vi "ClawGetStatus.vi"(8 "error in (no error)":errorcluster, 11 "MotorControlDevRef":T1={"DeviceStatus"={"status"=FALSE, "code"=0, "source"=""}, "Type"=enum."PWM", "PWM"={"Controller"=enum."Controller 1", "PWM Channel"=enum."PWM 1", "DeadBand"={"Name"="", "maxPositivePwm"=0, "minPositivePwm"=0, "centerPwm"=0, "maxNegativePwm"=0, "minNegativePwm"=0, "angularRange"=0}}, "CAN"={"Device Number"=0, "Control Mode"=enum."Percent VBus", "Semaphore"=refnum, "Max Vout"=12.0, "TalonSRX Control Mode"=enum."Percent VBus"}, "Invert"=FALSE, "TransformRef"=refnum, "InvTransformRef"=refnum}) -> (0 "error out":errorcluster, 1 "Holding Bin":bool, 2 "Claw State":enum16{"Open", "Closed", "Neither"}(ring), 3 "MotorControlDevRef":T1={"DeviceStatus"={"status"=FALSE, "code"=0, "source"=""}, "Type"=enum."PWM", "PWM"={"Controller"=enum."Controller 1", "PWM Channel"=enum."PWM 1", "DeadBand"={"Name"="", "maxPositivePwm"=0, "minPositivePwm"=0, "centerPwm"=0, "maxNegativePwm"=0, "minNegativePwm"=0, "angularRange"=0}}, "CAN"={"Device Number"=0, "Control Mode"=enum."Percent VBus", "Semaphore"=refnum, "Max Vout"=12.0, "TalonSRX Control Mode"=enum."Percent VBus"}, "Invert"=FALSE, "TransformRef"=refnum, "InvTransformRef"=refnum}, 5 "Claw Angle":dbl)   [LabVIEW 2014]
uses:
  <vilib>/Rock Robotics/WPI/MotorControl/WPI_MotorControlDeviceRef.ctl
  <vilib>/Rock Robotics/WPI/MotorControl/WPI_MotorControlType.ctl
  <vilib>/Rock Robotics/SystemInterfaces/Typedef/FPGA_TypedefDigitalModule.ctl
  <vilib>/Rock Robotics/SystemInterfaces/DIO/FPGA_DIOPWMChannel.ctl
  <vilib>/Rock Robotics/WPI/PWM/WPI_PWMDeadband.ctl
  <vilib>/Rock Robotics/WPI/CAN/Jaguar/SubVIs/WPI_CANJaguar_ControlMode.ctl
  <vilib>/Rock Robotics/WPI/CAN/TalonSRX/WPI_CANTalonSRX_APIControlMode.ctl
  <vilib>/Rock Robotics/WPI/PWM/WPI_PWMTransform_ConPane.ctl
  Robot Global Data.vi
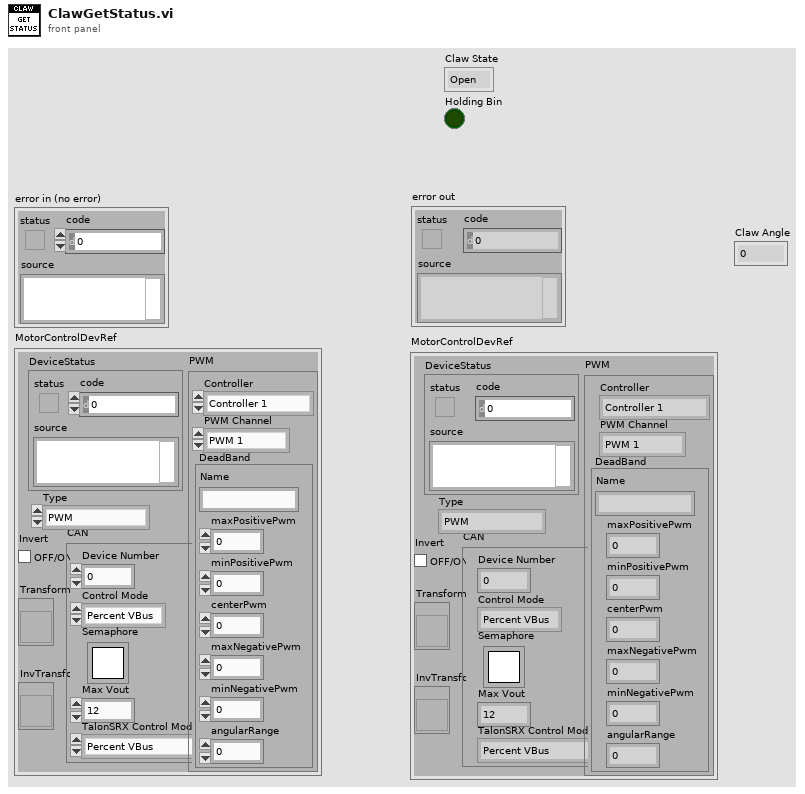
[diagram p1: front panel]
types:
  T1 = typedef "WPI_MotorControlDeviceRef.ctl" = cluster{"DeviceStatus":errorcluster, "Type":T2, "PWM":cluster{"Controller":T3, "PWM Channel":T4, "DeadBand":T5}, "CAN":cluster{"Device Number":u8, "Control Mode":T6, "Semaphore":T7, "Max Vout":dbl, "TalonSRX Control Mode":T8}, "Invert":bool, "TransformRef":T9, "InvTransformRef":T9}
  T2 = typedef "WPI_MotorControlType.ctl" = enum16{"PWM", "CAN", "CANTalonSRX"}
  T3 = typedef "FPGA_TypedefDigitalModule.ctl" = enum16{"Controller 1"}
  T4 = typedef "FPGA_DIOPWMChannel.ctl" = enum8{"PWM 0", "PWM 1", "PWM 2", "PWM 3", "PWM 4", "PWM 5", "PWM 6", "PWM 7", "PWM 8", "PWM 9", "PWM MXP 0", "PWM MXP 1", "PWM MXP 2", "PWM MXP 3", "PWM MXP 4", "PWM MXP 5", "PWM MXP 6", "PWM MXP 7", "PWM MXP 8", "PWM MXP 9", "Invalid"}
  T5 = typedef "WPI_PWMDeadband.ctl" = cluster{"Name":string, "maxPositivePwm":i32, "minPositivePwm":i32, "centerPwm":i32, "maxNegativePwm":i32, "minNegativePwm":i32, "angularRange":u16}
  T6 = typedef "WPI_CANJaguar_ControlMode.ctl" = enum8{"Percent VBus", "Current", "Speed", "Position", "Voltage"}
  T7 = typedef "Semaphore RefNum" = refnum<k1>
  T8 = typedef "WPI_CANTalonSRX_APIControlMode.ctl" = enum8{"Percent VBus", "Speed", "Position", "Slave", "Unchanged / Invalid"}
  T9 = typedef "WPI_PWMTransform_ConPane.ctl" = refnum<vi>
  T10 = typedef "WPI_CANTalonSRX_GlobalStatus.ctl" = cluster{"Applied Throttle":dbl, "Module Enabled":bool, "CAN Error":errorcluster, "Closed Loop Error":dbl, "Forward Limit Switch Closed":bool, "Reverse Limit Switch Closed":bool, "Sensor Position":dbl, "Sensor Velocity":dbl, "Current":dbl, "Sticky Fault - Over Temp":bool, "Sticky Fault - Under Voltage":bool, "Sticky Fault - Forward Limit":bool, "Sticky Fault - Reverse Limit":bool, "Sticky Fault - Forward Soft Limit":bool, "Sticky Fault - Reverse Soft Limit":bool, "Brake is Enabled":bool, "Encoder Position":dbl, "Encoder Velocity":dbl, "Encoder Index Count":dbl, "Encoder A Pin State":bool, "Encoder B Pin State":bool, "Encoder Index Pin State":bool, "Analog In":dbl, "Analog In Velocity":dbl, "Temperature (C)":dbl, "Battery Voltage":dbl}
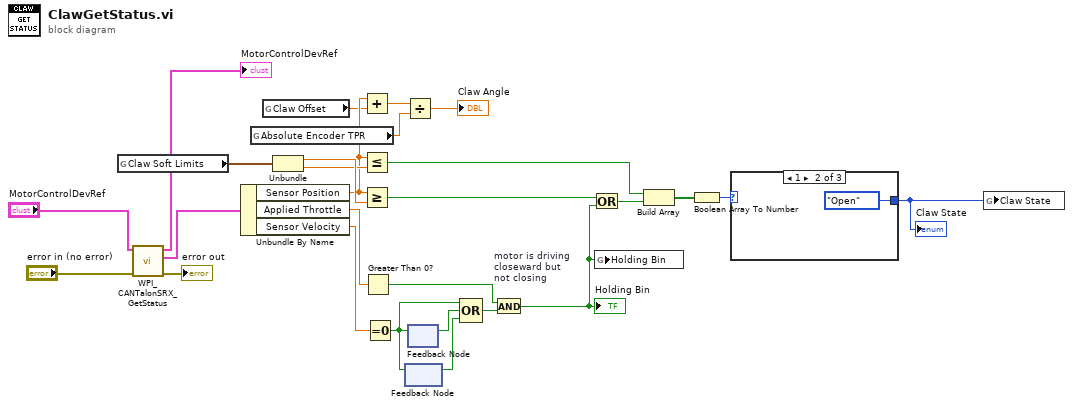
[diagram p0: block diagram]
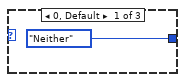
[diagram p2: hidden frame]
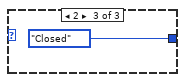
[diagram p3: hidden frame]
diagram:
  n1 = global read "Robot Global Data.vi" "Claw Soft Limits"() -> (w26:cluster{"Forward":dbl, "Reverse":dbl})
  n2 = call <vilib>:"WPI_CANTalonSRX_GetStatus.vi"("error in (no error)"="error in (no error)", "CAN Talon SRX Ref"="MotorControlDevRef") -> ("error out"=→"error out":errorcluster, "Talon SRX Status"=w27:T10, "CAN Talon SRX Ref Out"=→"MotorControlDevRef":T1)  [unwired: 7 in]
  n3 = Unbundle By Name(w27) -> ("Sensor Position"=w23:dbl, "Applied Throttle"=w7:dbl, "Sensor Velocity"=w5:dbl)
  n4 = global read "Robot Global Data.vi" "Absolute Encoder TPR"() -> (w16:dbl)
  n5 = global read "Robot Global Data.vi" "Claw Offset"() -> (w18:dbl)
  n6 = Unbundle(w26) -> ("Forward"=w25:dbl, "Reverse"=w24:dbl)
  n7 = Add(x=w23, y=w18) -> (x+y=w17:dbl)
  n8 = Less Or Equal?(x=w23, y=w24) -> (x <= y?=w11:bool)
  n9 = Greater Or Equal?(x=w23, y=w25) -> (x >= y?=w9:bool)
  n10 = Greater Than 0?(x=w7) -> (x > 0?=w8:bool)
  n11 = Equal To 0?(x=w5) -> (x = 0?=w4:bool)
  n12 = Divide(x=w17, y=w16) -> (x/y=→"Claw Angle":dbl)
  n13 = feedback #1() -> (w2:bool)  [unwired: 1 in]
  n14 = feedback-in #1(w4) -> ()
  n15 = feedback-in #2(w4) -> ()
  n16 = feedback #2() -> (w3:bool)  [unwired: 1 in]
  n17 = Compound Arithmetic op=OR(w4, w3, w2) -> (w1:bool)
  n18 = And "motor is driving\ncloseward but\nnot closing"(x=w8, y=w1) -> (x .and. y?=w6:bool)
  "Holding Bin" <- w6
  n19 = Or(x=w9, y=w6) -> (x .or. y?=w10:bool)
  n20 = global write "Robot Global Data.vi" "Holding Bin"(w6) -> ()
  n21 = Build Array(w11, w10) -> (w13:bool[])
  n22 = Boolean Array To Number(Boolean array=w13) -> (number=w12:u32)
  n23 = case shown="1" w12 {
    tunnel: [enum16{"Open", "Closed", "Neither"}."Neither" ("Claw State") enum16{"Open", "Closed", "Neither"}."Open" ("Claw State") enum16{"Open", "Closed", "Neither"}."Closed" ("Claw State")] -> w14
    frame 0, Default {
    }
    frame 1 {
    }
    frame 2 {
    }
  }
  "Claw State" <- w14
  n24 = global write "Robot Global Data.vi" "Claw State"(w14) -> ()
